vi "Read_binary.vi"() -> ()   [LabVIEW 2015]
panel:
  out "Waveform Graph":i16[](graph)
  out "error out":errorcluster
  in  "Path":path=path "C:/GitHub/PulseEcho/Data/TestData/data.bin"
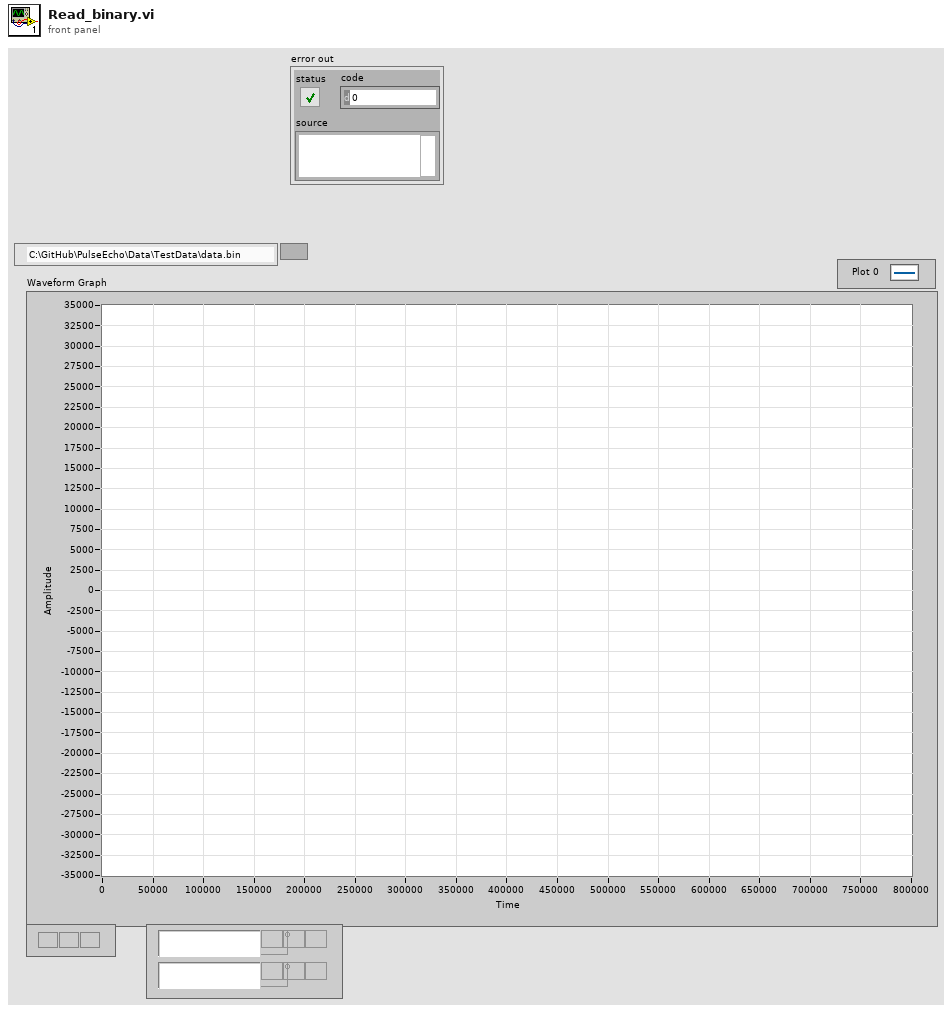
[diagram p1: front panel]
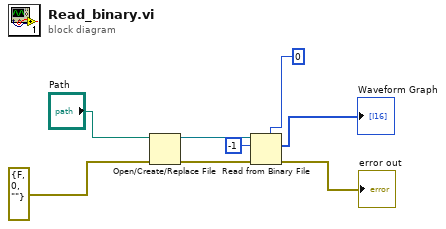
[diagram p0: block diagram]
diagram:
  n1 = Open/Create/Replace File(file path (use dialog)="Path", error in=errorcluster {"status"=FALSE, "code"=0, "source"=""}) -> (refnum out=w3:refnum<file>, error out=w7:errorcluster)  [unwired: 4 in, 1 out]
  n2 = Read from Binary File(5:i16 0, 8:w7, 10:-1 ("count (1)"), 11:w3) -> (0:→"error out":errorcluster, 2:→"Waveform Graph":i16[])  [unwired: 2 in, 2 out]
